vi "Initialize Shared Variable Channel Data.vi"(11 "Channel Refs in":T2[](array[typedef]) format="%.0x") -> (3 "Shared Variable Channel Data":T1 {"Channel Refs" format="%.0x"})   [LabVIEW 2012, in "Shared Variable Custom Device.lvlib"]
uses:
  Shared Variable Custom Device.lvlib
  <vilib>/NI Veristand/Custom Device API/Custom Device Item Ref.ctl
  Channel Information Control.ctl
  <vilib>/NI Veristand/Custom Device API/Custom Device API.lvlib
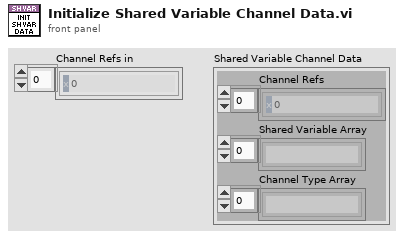
[diagram p1: front panel]
types:
  T1 = typedef "Shared Variable Custom Device.lvlib/Channel Information Control.ctl" = cluster{"Channel Refs":T2[], "Shared Variable Array":string[], "Channel Type Array":string[]}
  T2 = typedef "Custom Device API.lvlib/Custom Device Item Ref.ctl" = u64
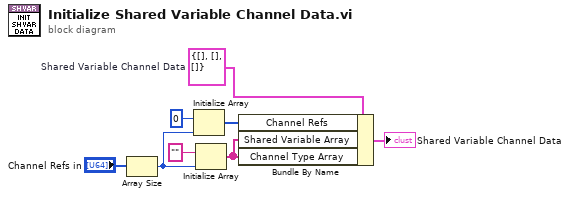
[diagram p0: block diagram]
diagram:
  w1 = T1 {"Channel Refs"=[], "Shared Variable Array"=[], "Channel Type Array"=[]}  # Shared Variable Channel Data
  n1 = Array Size(array="Channel Refs in") -> (size(s)=w6:i32)
  n2 = Initialize Array(T2 0 ("Section Ref in"), w6) -> (w5:T2[])
  n3 = Initialize Array("", w6) -> (w8:string[])
  n4 = Bundle By Name(cluster=w1, "Channel Refs"=w5, "Shared Variable Array"=w8, "Channel Type Array"=w8) -> (→"Shared Variable Channel Data":T1)
